vi "Read Listener NQR.vi"(11 "Unregistration Msg In":refnum<class "Unregistration Msg.lvclass">) -> (2 "subscriber NQR":refnum<class "Message Enqueuer.lvclass">, 3 "Unregistration Msg Out":refnum<class "Unregistration Msg.lvclass">)   [LabVIEW 2016, in "Data Broadcasting.lvlib" / "Unregistration Msg.lvclass"]
doc: "-------------\nCopyright (c) 2013, Staab Engineering, a Texas Limited Liability Company\nAll rights reserved.\n\nRedistribution and use in source and binary forms, with or without modification, are permitted provided that the following conditions are met:\n\n1. Redistributions of source code must retain the above copyright notice, this list of conditions and the following disclaimer.\n2. Redistributions in binary form must reproduce the above copyright notice, this list of conditions and the following disclaimer in the documentation and/or other materials provided with the distribution.\n\nTHIS SOFTWARE IS PROVIDED BY THE COPYRIGHT HOLDERS AND CONTRIBUTORS \"AS IS\" AND ANY EXPRESS OR IMPLIED WARRANTIES, INCLUDING, BUT NOT LIMITED TO, THE IMPLIED WARRANTIES OF MERCHANTABILITY AND FITNESS FOR A PARTICULAR PURPOSE ARE DISCLAIMED. IN NO EVENT SHALL THE COPYRIGHT HOLDER OR CONTRIBUTORS BE LIABLE FOR ANY DIRECT, INDIRECT, INCIDENTAL, SPECIAL, EXEMPLARY, OR CONSEQUENTIAL DAMAGES (INCLUDING, BUT NOT LIMITED TO, PROCUREMENT OF SUBSTITUTE GOODS OR SERVICES; LOSS OF USE, DATA, OR PROFITS; OR BUSINESS INTERRUPTION) HOWEVER CAUSED AND ON ANY THEORY OF LIABILITY, WHETHER IN CONTRACT, STRICT LIABILITY, OR TORT (INCLUDING NEGLIGENCE OR OTHERWISE) ARISING IN ANY WAY OUT OF THE USE OF THIS SOFTWARE, EVEN IF ADVISED OF THE POSSIBILITY OF SUCH DAMAGE."
uses:
  <userlib>/_Frameworks/Staab/AF Data Broadcasting/Data Broadcasting/Unregistration Msg/Unregistration Msg.lvclass
  <vilib>/ActorFramework/Message Enqueuer/Message Enqueuer.lvclass
  <userlib>/_Frameworks/Staab/AF Data Broadcasting/Data Broadcasting/Unregistration Msg/Unregistration Msg.lvclass/Unregistration Msg.ctl
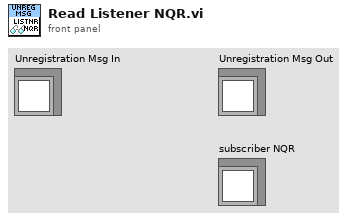
[diagram p1: front panel]
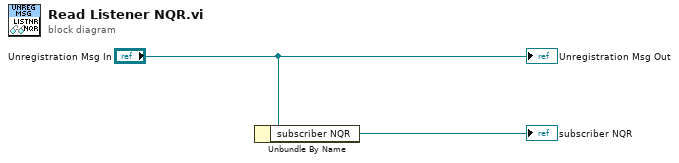
[diagram p0: block diagram]
diagram:
  n1 = Unbundle By Name("Unregistration Msg In") -> ("subscriber NQR"=→"subscriber NQR":refnum<class "Message Enqueuer.lvclass">)
  "Unregistration Msg Out" <- "Unregistration Msg In"
